vi "test_resample_fixed.vi"() -> ()   [LabVIEW 2013]
uses:
  <vilib>/measure/maspectr.llb/Power Spectrum and PSD Export Mode.ctl
  <vilib>/measure/maspectr.llb/FFT Power Spectrum and PSD for 1 Chan.vi
  <vilib>/Analysis/2dsp.llb/Resample (constant to constant,single -channel).vi
  <vilib>/measure/NI_MAPro.lvlib
  <vilib>/Analysis/NI_AALPro.lvlib
panel:
  out "Waveform Graph 2":i16[](graph)
  out "size(s) 2":i32
  out "Waveform Graph":dbl[](graph)
  out "size(s)":i32
  out "power spectrum 2":cluster{"f0":dbl, "df":dbl, "magnitude":dbl[]}(graph)
  out "power spectrum":cluster{"f0":dbl, "df":dbl, "magnitude":dbl[]}(graph)
  in  "Ring":u16(ring) items=["125 MHz", "375 MHz"]
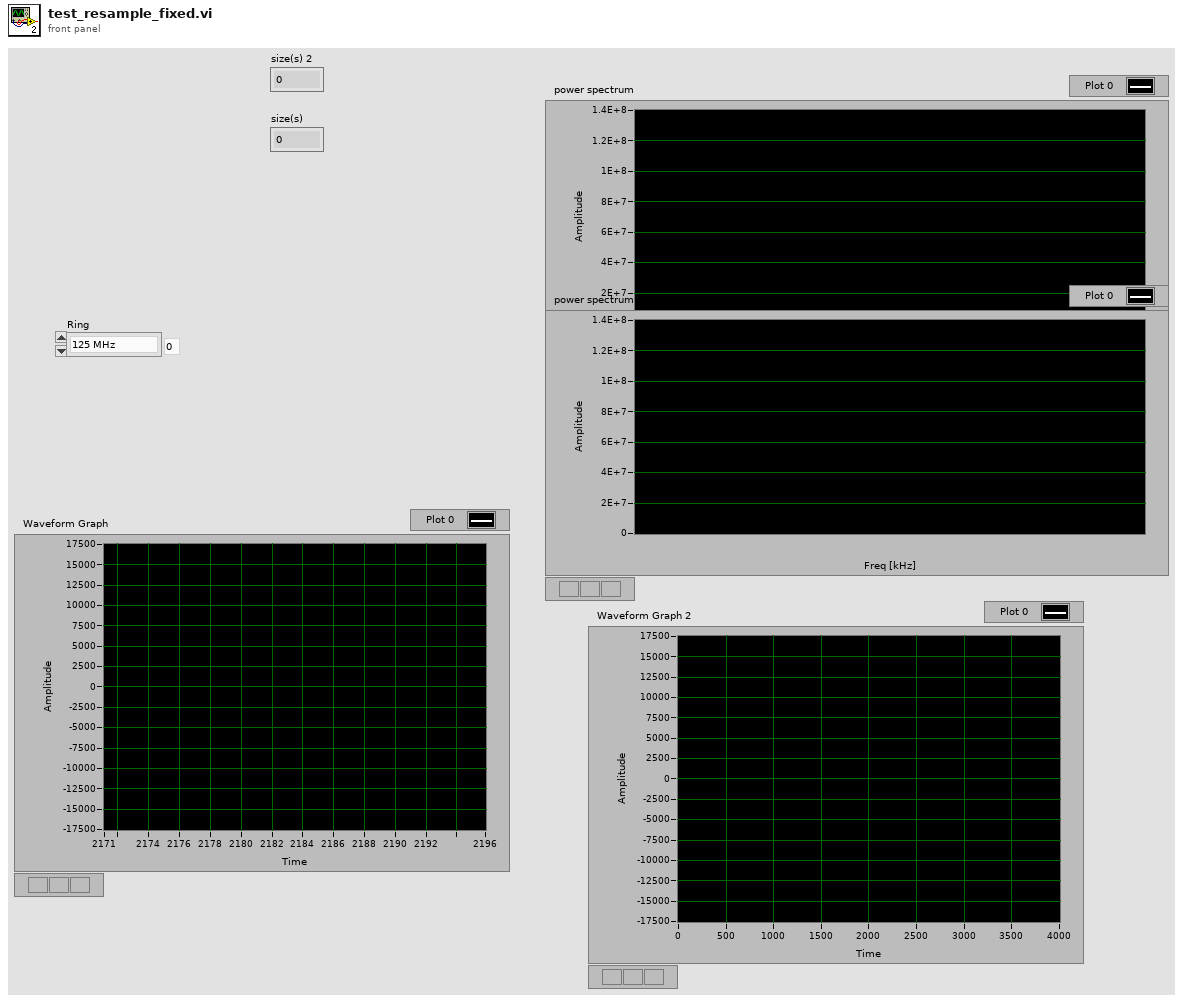
[diagram p1: front panel]
types:
  T1 = typedef "NI_MAPro.lvlib/Power Spectrum and PSD Export Mode.ctl" = u16
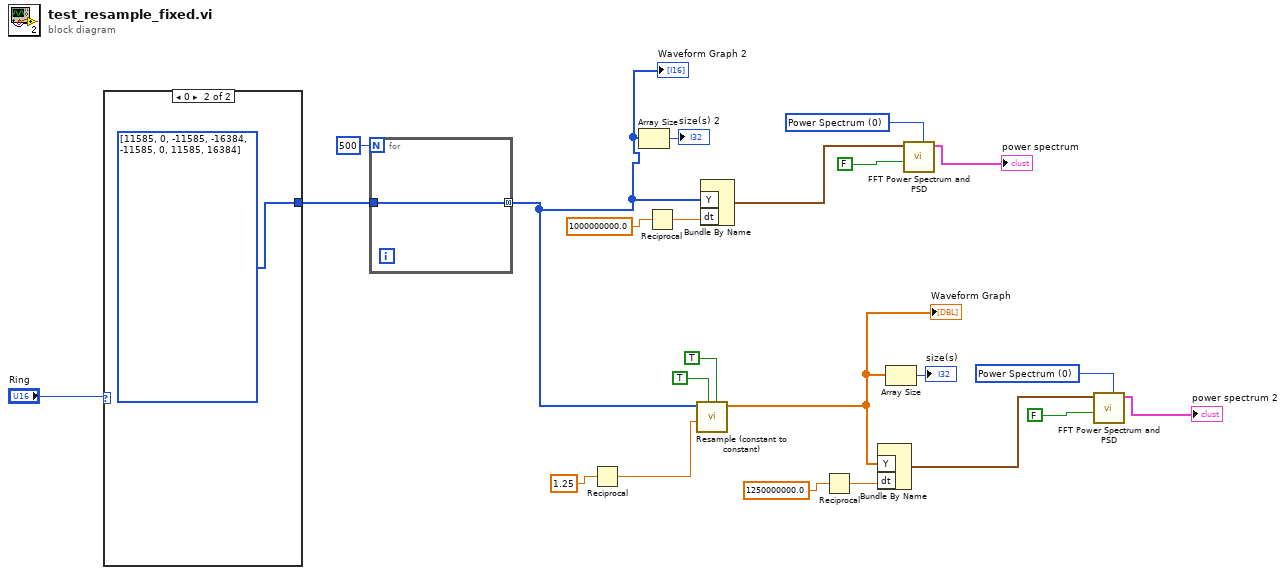
[diagram p0: block diagram]
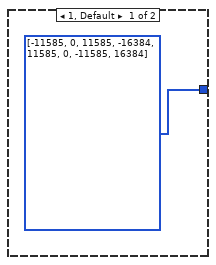
[diagram p2: hidden frame]
diagram:
  w6 = T1 0 items=["Power Spectrum", "Power Spectral Density"] ("export mode")
  w20 = T1 0 items=["Power Spectrum", "Power Spectral Density"] ("export mode")
  n1 = case shown="0" "Ring" {
    tunnel: [i16[] [-11585, 0, 11585, -16384, 11585, 0, -11585, 16384] ("output array 2") i16[] [11585, 0, -11585, -16384, -11585, 0, 11585, 16384] ("output array 2")] -> w21
    frame 1, Default {
    }
    frame 0 {
    }
  }
  n2 = for {
    N: 500 -> [_]
    tunnel: [w26] -> w1 mode=concatenating
    tunnel: w21 -> [w26]
  }
  "Waveform Graph 2" <- w1
  n3 = Reciprocal(x=1.25 ("dt")) -> (1/x=w13:dbl)
  n4 = Array Size(array=w1) -> (size(s)=→"size(s) 2":i32)
  n5 = Reciprocal(x=1000000000.0 ("dt")) -> (1/x=w16:dbl)
  n6 = call-poly <vilib>:"Resample (constant to constant).vi"("anti-aliasing?"=TRUE, "reset?"=TRUE, "dt"=w13, "X"=w1) -> ("Y"=w3:dbl[])  [unwired: 5 in, 2 out]
  "Waveform Graph" <- w3
  n7 = Bundle By Name("Y"=w1, "dt"=w16) -> (w19:waveform(i16))  [unwired: 1 in]
  n8 = Reciprocal(x=1250000000.0 ("dt")) -> (1/x=w10:dbl)
  n9 = Bundle By Name("Y"=w3, "dt"=w10) -> (w5:waveform(dbl))  [unwired: 1 in]
  n10 = Array Size(array=w3) -> (size(s)=→"size(s)":i32)
  n11 = call-poly <vilib>:"FFT Power Spectrum and PSD.vi"("export mode"=w20, "dB On (F)"=FALSE, "time signal"=w19) -> ("Power Spectrum / PSD"=→"power spectrum":cluster{"f0":dbl, "df":dbl, "magnitude":dbl[]})  [unwired: 5 in, 3 out]
  n12 = call-poly <vilib>:"FFT Power Spectrum and PSD.vi"("export mode"=w6, "dB On (F)"=FALSE, "time signal"=w5) -> ("Power Spectrum / PSD"=→"power spectrum 2":cluster{"f0":dbl, "df":dbl, "magnitude":dbl[]})  [unwired: 5 in, 3 out]
